vi "Drive_Teleop.vi"(10 "Control_Cluster":T1) -> ()   [LabVIEW 2019]
uses:
  Subsystems/Drive_Globals.vi
  Subsystems/Drive/DriveSetCluster.ctl
  Utility_VIs/Joystick_Controls.ctl
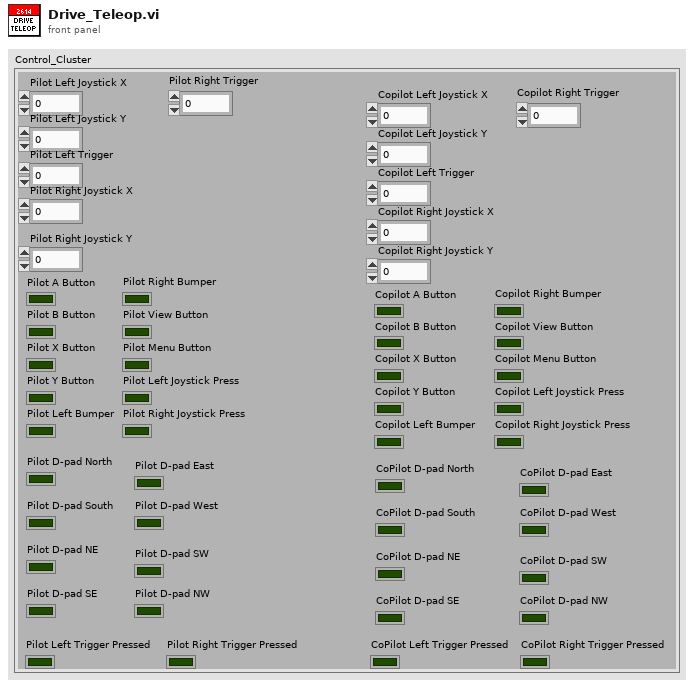
[diagram p1: front panel]
types:
  T1 = typedef "Joystick_Controls.ctl" = cluster{"Pilot Left Joystick X":dbl, "Pilot Left Joystick Y":dbl, "Pilot A Button":bool, "Pilot B Button":bool, "Pilot X Button":bool, "Pilot Y Button":bool, "Pilot Left Bumper":bool, "Pilot Right Bumper":bool, "Pilot View Button":bool, "Pilot Menu Button":bool, "Pilot Left Joystick Press":bool, "Pilot Right Joystick Press":bool, "Pilot Left Trigger":dbl, "Pilot Right Joystick X":dbl, "Pilot Right Joystick Y":dbl, "Pilot Right Trigger":dbl, "Copilot Left Joystick X":dbl, "Copilot Left Joystick Y":dbl, "Copilot A Button":bool, "Copilot B Button":bool, "Copilot X Button":bool, "Copilot Y Button":bool, "Copilot Left Bumper":bool, "Copilot Right Bumper":bool, "Copilot View Button":bool, "Copilot Menu Button":bool, "Copilot Left Joystick Press":bool, "Copilot Right Joystick Press":bool, "Copilot Left Trigger":dbl, "Copilot Right Joystick X":dbl, "Copilot Right Joystick Y":dbl, "Copilot Right Trigger":dbl, "Pilot D-pad North":bool, "Pilot D-pad South":bool, "Pilot D-pad East":bool, "Pilot D-pad West":bool, "Pilot D-pad NE ":bool, "Pilot D-pad SE":bool, "Pilot D-pad SW":bool, "Pilot D-pad NW":bool, "CoPilot D-pad North":bool, "CoPilot D-pad South":bool, "CoPilot D-pad East":bool, "CoPilot D-pad West":bool, "CoPilot D-pad NE":bool, "CoPilot D-pad SE":bool, "CoPilot D-pad SW":bool, "CoPilot D-pad NW":bool, "Pilot Left Trigger Pressed":bool, "Pilot Right Trigger Pressed":bool, "CoPilot Left Trigger Pressed":bool, "CoPilot Right Trigger Pressed":bool}
  T2 = typedef "DriveSetCluster.ctl" = cluster{"Front/Back":dbl, "Turn":dbl, "Speed_Control?":bool}
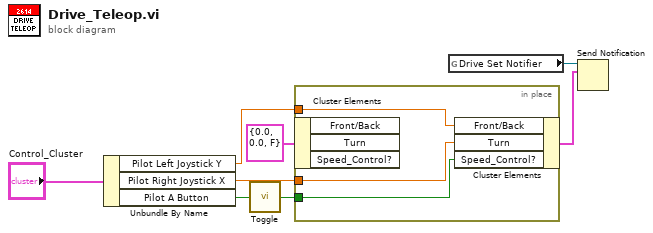
[diagram p0: block diagram]
diagram:
  n1 = Unbundle By Name("Control_Cluster") -> ("Pilot Left Joystick Y"=w3:dbl, "Pilot Right Joystick X"=w2:dbl, "Pilot A Button"=w8:bool)
  n2 = call "Toggle.vi"("Boolean"=w8) -> ("Boolean Out"=w1:bool)
  n3 = in-place {
    in-place-border: w3 -> [w11]
    in-place-border: w2 -> [w10]
    in-place-border: w1 -> [w9]
    n4 = in-place-cluster #1(T2 {"Front/Back"=0.0, "Turn"=0.0, "Speed_Control?"=FALSE} ("Drive Set Cluster")) -> ()  [unwired: 3 out]
    n5 = in-place-cluster #1("Front/Back"=w11, "Turn"=w10, "Speed_Control?"=w9) -> (w4:T2)
  }
  n6 = global read "Drive_Globals.vi" "Drive Set Notifier"() -> (w7:refnum<notifier>)
  n7 = Send Notification(notification=w4, notifier=w7) -> ()  [unwired: 1 in, 2 out]
